vi "CallArm.vi"(6 "Time out?":u8, 8 "error in (no error)":errorcluster, 11 "FPGA VI引用输入":refnum<k20>) -> (0 "error out":errorcluster, 3 "FPGA VI引用输出":refnum<k20>)   [LabVIEW 2015]
uses:
  <vilib>/Utility/error.llb/Error Cluster From Error Code.vi
  <vilib>/rvi/errors/niLvFpgaAdjustHostInterfaceError.vi
  <vilib>/rvi/interface/nirviReadWriteControl/nirviReadWriteControl.xnode
  NiFpgaLv.dll
  <vilib>/rvi/interface/Simulation/niFpgaSimulationCallBeginRW.vi
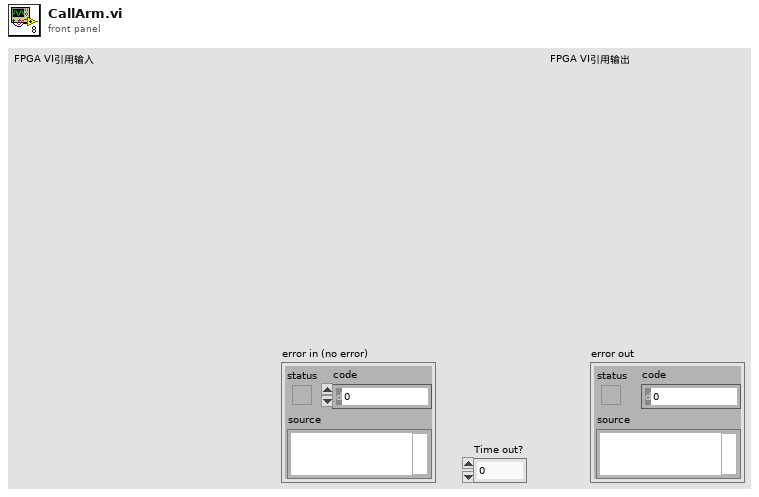
[diagram p1: front panel]
types:
  T1 = enum8{"IDLE", "SetIDLE", "Config", "Arm", "Read", "Write", "AutoRead"}
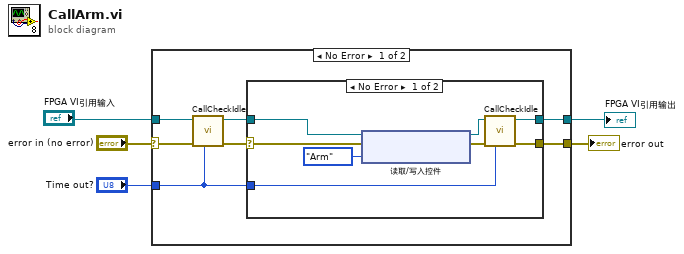
[diagram p0: block diagram]
diagram:
  n1 = case shown="No Error" "error in (no error)" {
    selector: "error in (no error)" -> [w11 w24]
    tunnel: [w12 w24] -> w5
    tunnel: "Time out?" -> [w9 _]
    tunnel: "FPGA VI引用输入" -> [w6 w23]
    tunnel: [w7 w23] -> w1
    frame No Error {
      n2 = call "CallCheckIdle.vi"("Time out?"=w9, "error in (no error)"=w11, "FPGA VI引用输入"=w6) -> ("error out"=w10:errorcluster, "FPGA VI引用输出"=w8:refnum<k20>)  [unwired: 7 in]
      n3 = case shown="No Error" w10 {
        selector: w10 -> [w20 w22]
        tunnel: [w17 w22] -> w12
        tunnel: w9 -> [w15 _]
        tunnel: w8 -> [w19 w21]
        tunnel: [w13 w21] -> w7
        frame No Error {
          n4 = xnode "读取/写入控件"("FPGA VI Reference In"=w19, "error in"=w20, "ProtocolControl"=T1."Arm") -> ("FPGA VI Reference Out"=w14:refnum<k20>, "error out"=w16:errorcluster)
          n5 = call "CallCheckIdle.vi"("Time out?"=w15, "error in (no error)"=w16, "FPGA VI引用输入"=w14) -> ("error out"=w17:errorcluster, "FPGA VI引用输出"=w13:refnum<k20>)  [unwired: 7 in]
        }
        frame Error {
        }
      }
    }
    frame Error {
    }
  }
  "error out" <- w5
  "FPGA VI引用输出" <- w1
